vi "PixyGetObject.vi"(11 "Input Frame":string) -> (0 "Remainder of Frame":string, 3 "Object":string, 5 "Empty?":bool)   [LabVIEW 2016]
uses:
  <vilib>/regexp/Match Regular Expression.xnode
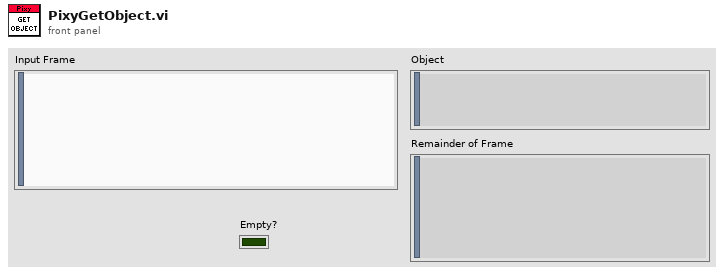
[diagram p1: front panel]
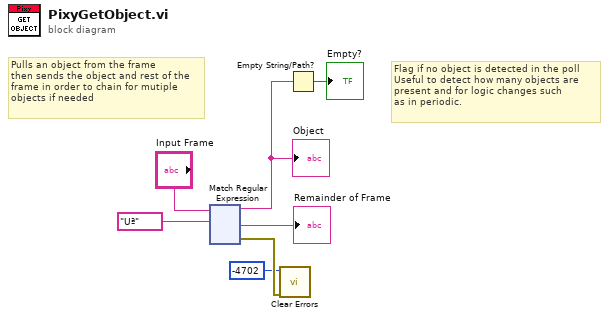
[diagram p0: block diagram]
diagram:
  # "Flag if no object is detected in the poll\nUseful to detect how many objects are \npresent and for logic changes such\nas in periodic."
  # "Pulls an object from the frame\nthen sends the object and rest of the\nframe in order to chain for mutiple\nobjects if needed"
  n1 = xnode "Match Regular Expression"("input string"="Input Frame", "regular expression"="Uª") -> ("before match"=w3:string, "after match"=→"Remainder of Frame":string, "error out"=w2:errorcluster)  [unwired: 4 in, 2 out]
  "Object" <- w3
  n2 = call <vilib>:"Clear Errors.vi"("error in (no error)"=w2, "specific error code to clear (0: all)"=-4702) -> ()  [unwired: 4 in, 2 out]
  n3 = Empty String/Path?(string/path=w3) -> (empty?=→"Empty?":bool)
